vi "Cleanup.vi"(8 "error in (no error)":errorcluster, 11 "Stop Under Body Wash in":refnum<class "Stop Under Body Wash.lvclass">) -> (0 "error out":errorcluster, 3 "Stop Under Body Wash out":refnum<class "Stop Under Body Wash.lvclass">)   [LabVIEW 2019, in "Stop Under Body Wash.lvclass"]
uses:
  <vilib>/gpm_packages/@cs/Car-wash/Source/Process Steps/Stop Under Body Wash/Stop Under Body Wash.lvclass
  <vilib>/gpm_packages/@cs/Car-wash/Source/iProcess Step Model/iProcess Step Model/iProcess Step Model.lvclass
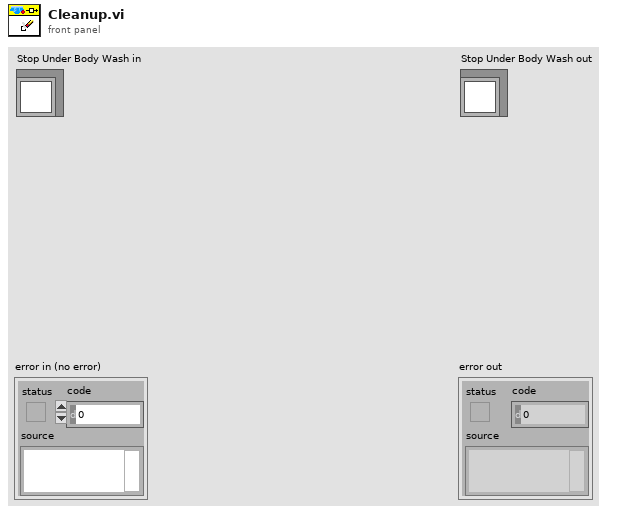
[diagram p1: front panel]
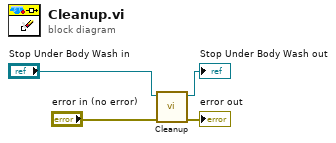
[diagram p0: block diagram]
diagram:
  n1 = call-parent "Cleanup.vi"("error in (no error)"="error in (no error)", "iProcess Step Model in"="Stop Under Body Wash in") -> ("error out"=→"error out":errorcluster, "iProcess Step Model out"=→"Stop Under Body Wash out":refnum<class "Stop Under Body Wash.lvclass">)  [unwired: 8 in]
